vi "Configure Smoothing.vi"(6 "Smoothing Aperture (1.5 %)":dbl=1.5 format="%^#_9g", 7 "Enable Smoothing (Disable)":bool, 8 "error in (no error)":errorcluster, 9 "Select Trace (1: 1)":u16(ring)=1 items=["1"=1, "2"=2, "3"=3, "4"=4, "5"=5, "6"=6, "7"=7, "8"=8], 10 "Measurement Type (6: Phase Noise)":u16(ring)=6 items=["AM Noise"=1, "Baseband Noise"=2, "Freq/Power"=3, "Spectrum"=4, "Transient"=5, "Phase Noise"=6, "User"=7], 11 "VISA resource name":refnum<visa-resource-name>) -> (0 "error out":errorcluster, 3 "VISA resource name out":refnum<visa-resource-name>)   [LabVIEW 2011, in "Agilent E5052X.lvlib"]
doc: "Configures the instrument to apply smoothing to all types of measurement data.\n\n<b>Note: </b>\n\n\"Configure Measurement Characteristics\" VI must be run before this VI."
uses:
  Agilent E5052X.lvlib
panel:
  # "Smoothing Settings"
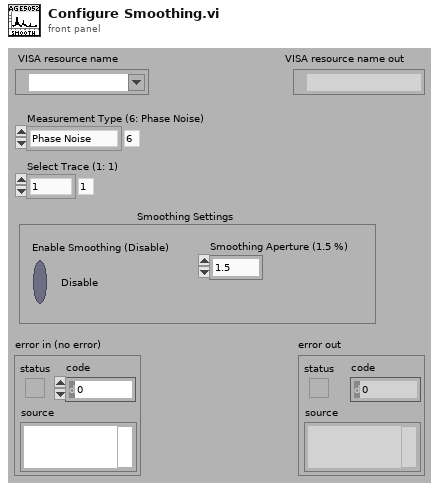
[diagram p1: front panel]
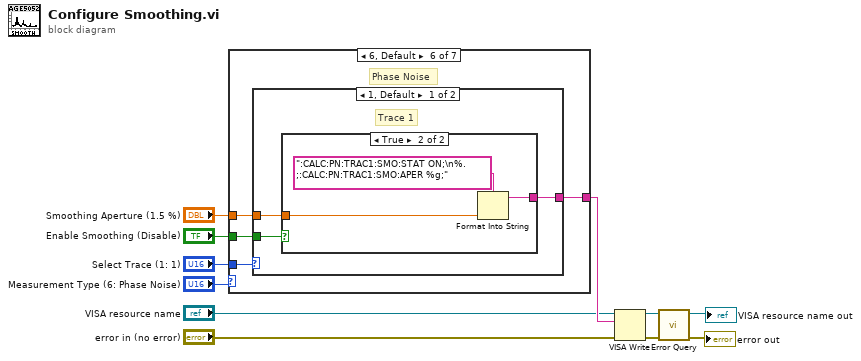
[diagram p0: block diagram]
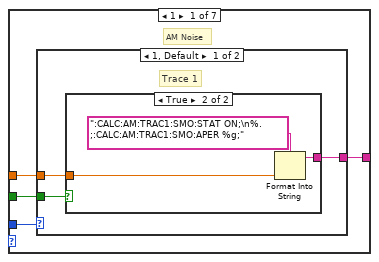
[diagram p2: hidden frame]
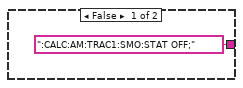
[diagram p3: hidden frame]
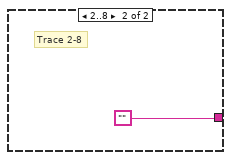
[diagram p4: hidden frame]
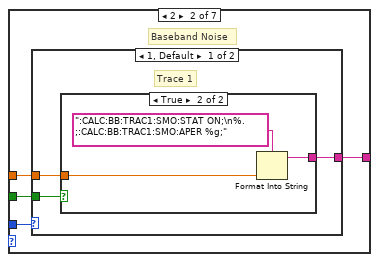
[diagram p5: hidden frame]
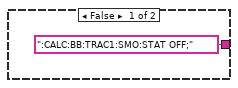
[diagram p6: hidden frame]
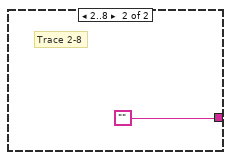
[diagram p7: hidden frame]
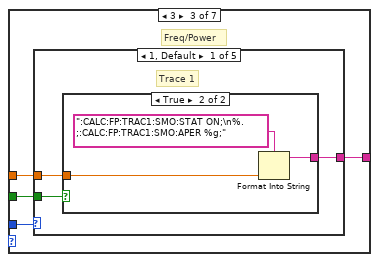
[diagram p8: hidden frame]
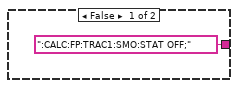
[diagram p9: hidden frame]
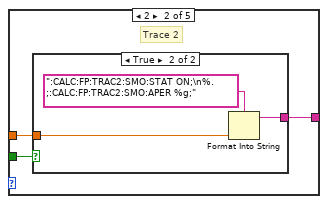
[diagram p10: hidden frame]
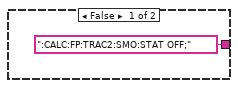
[diagram p11: hidden frame]
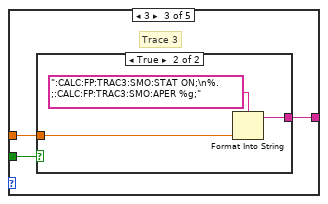
[diagram p12: hidden frame]
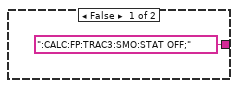
[diagram p13: hidden frame]
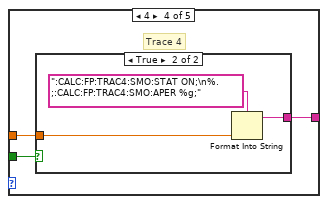
[diagram p14: hidden frame]
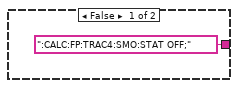
[diagram p15: hidden frame]
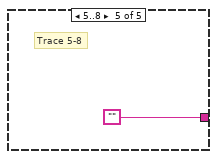
[diagram p16: hidden frame]
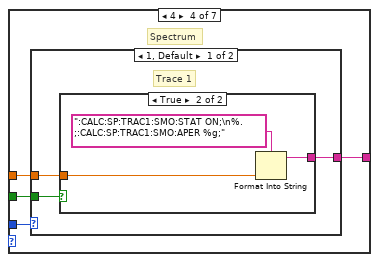
[diagram p17: hidden frame]
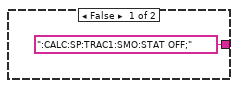
[diagram p18: hidden frame]
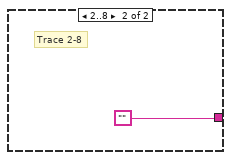
[diagram p19: hidden frame]
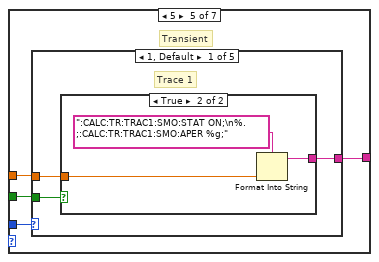
[diagram p20: hidden frame]
diagram:
  n1 = case shown="6, Default" "Measurement Type (6: Phase Noise)" {
    tunnel: "Enable Smoothing (Disable)" -> [w14 w26 w38 w71 w83 w116 w128]
    tunnel: "Select Trace (1: 1)" -> [w15 w25 w37 w70 w82 w115 w127]
    tunnel: "Smoothing Aperture (1.5 %)" -> [w13 w27 w39 w72 w84 w117 w129]
    tunnel: [w12 w24 w36 w69 w81 w114 w126] -> w6
    frame 1 {
      # "AM Noise"
      n2 = case shown="1, Default" w15 {
        tunnel: w14 -> [w18 _]
        tunnel: w13 -> [w17 _]
        tunnel: [w16 ""] -> w12
        frame 1, Default {
          # "Trace 1"
          n3 = case shown="True" w18 {
            tunnel: w17 -> [_ w22]
            tunnel: [":CALC:AM:TRAC1:SMO:STAT OFF;" w20] -> w16
            frame False {
            }
            frame True {
              n4 = Format Into String(format string=":CALC:AM:TRAC1:SMO:STAT ON;\n%.;:CALC:AM:TRAC1:SMO:APER %g;", w22) -> (resulting string=w20:string)  [unwired: 2 in, 1 out]
            }
          }
        }
        frame 2..8 {
          # "Trace 2-8"
        }
      }
    }
    frame 2 {
      # "Baseband Noise"
      n5 = case shown="1, Default" w25 {
        tunnel: w26 -> [w30 _]
        tunnel: w27 -> [w29 _]
        tunnel: [w28 ""] -> w24
        frame 1, Default {
          # "Trace 1"
          n6 = case shown="True" w30 {
            tunnel: w29 -> [_ w34]
            tunnel: [":CALC:BB:TRAC1:SMO:STAT OFF;" w32] -> w28
            frame False {
            }
            frame True {
              n7 = Format Into String(format string=":CALC:BB:TRAC1:SMO:STAT ON;\n%.;:CALC:BB:TRAC1:SMO:APER %g;", w34) -> (resulting string=w32:string)  [unwired: 2 in, 1 out]
            }
          }
        }
        frame 2..8 {
          # "Trace 2-8"
        }
      }
    }
    frame 3 {
      # "Freq/Power"
      n8 = case shown="1, Default" w37 {
        tunnel: w38 -> [w42 w48 w55 w62 _]
        tunnel: w39 -> [w41 w49 w56 w63 _]
        tunnel: [w40 w47 w54 w61 ""] -> w36
        frame 1, Default {
          # "Trace 1"
          n9 = case shown="True" w42 {
            tunnel: w41 -> [_ w46]
            tunnel: [":CALC:FP:TRAC1:SMO:STAT OFF;" w44] -> w40
            frame False {
            }
            frame True {
              n10 = Format Into String(format string=":CALC:FP:TRAC1:SMO:STAT ON;\n%.;:CALC:FP:TRAC1:SMO:APER %g;", w46) -> (resulting string=w44:string)  [unwired: 2 in, 1 out]
            }
          }
        }
        frame 2 {
          # "Trace 2"
          n11 = case shown="True" w48 {
            tunnel: w49 -> [_ w53]
            tunnel: [":CALC:FP:TRAC2:SMO:STAT OFF;" w51] -> w47
            frame False {
            }
            frame True {
              n12 = Format Into String(format string=":CALC:FP:TRAC2:SMO:STAT ON;\n%.;:CALC:FP:TRAC2:SMO:APER %g;", w53) -> (resulting string=w51:string)  [unwired: 2 in, 1 out]
            }
          }
        }
        frame 3 {
          # "Trace 3"
          n13 = case shown="True" w55 {
            tunnel: w56 -> [_ w60]
            tunnel: [":CALC:FP:TRAC3:SMO:STAT OFF;" w58] -> w54
            frame False {
            }
            frame True {
              n14 = Format Into String(format string=":CALC:FP:TRAC3:SMO:STAT ON;\n%.;:CALC:FP:TRAC3:SMO:APER %g;", w60) -> (resulting string=w58:string)  [unwired: 2 in, 1 out]
            }
          }
        }
        frame 4 {
          # "Trace 4"
          n15 = case shown="True" w62 {
            tunnel: w63 -> [_ w67]
            tunnel: [":CALC:FP:TRAC4:SMO:STAT OFF;" w65] -> w61
            frame False {
            }
            frame True {
              n16 = Format Into String(format string=":CALC:FP:TRAC4:SMO:STAT ON;\n%.;:CALC:FP:TRAC4:SMO:APER %g;", w67) -> (resulting string=w65:string)  [unwired: 2 in, 1 out]
            }
          }
        }
        frame 5..8 {
          # "Trace 5-8"
        }
      }
    }
    frame 4 {
      # "Spectrum"
      n17 = case shown="1, Default" w70 {
        tunnel: w71 -> [w75 _]
        tunnel: w72 -> [w74 _]
        tunnel: [w73 ""] -> w69
        frame 1, Default {
          # "Trace 1"
          n18 = case shown="True" w75 {
            tunnel: w74 -> [_ w79]
            tunnel: [":CALC:SP:TRAC1:SMO:STAT OFF;" w77] -> w73
            frame False {
            }
            frame True {
              n19 = Format Into String(format string=":CALC:SP:TRAC1:SMO:STAT ON;\n%.;:CALC:SP:TRAC1:SMO:APER %g;", w79) -> (resulting string=w77:string)  [unwired: 2 in, 1 out]
            }
          }
        }
        frame 2..8 {
          # "Trace 2-8"
        }
      }
    }
    frame 5 {
      # "Transient"
      n20 = case shown="1, Default" w82 {
        tunnel: w83 -> [w87 w93 w100 w107 _]
        tunnel: w84 -> [w86 w94 w101 w108 _]
        tunnel: [w85 w92 w99 w106 ""] -> w81
        frame 1, Default {
          # "Trace 1"
          n21 = case shown="True" w87 {
            tunnel: w86 -> [_ w91]
            tunnel: [":CALC:TR:TRAC1:SMO:STAT OFF;" w89] -> w85
            frame False {
            }
            frame True {
              n22 = Format Into String(format string=":CALC:TR:TRAC1:SMO:STAT ON;\n%.;:CALC:TR:TRAC1:SMO:APER %g;", w91) -> (resulting string=w89:string)  [unwired: 2 in, 1 out]
            }
          }
        }
        frame 2 {
          # "Trace 2"
          n23 = case shown="True" w93 {
            tunnel: w94 -> [_ w98]
            tunnel: [":CALC:TR:TRAC2:SMO:STAT OFF;" w96] -> w92
            frame False {
            }
            frame True {
              n24 = Format Into String(format string=":CALC:TR:TRAC2:SMO:STAT ON;\n%.;:CALC:TR:TRAC2:SMO:APER %g;", w98) -> (resulting string=w96:string)  [unwired: 2 in, 1 out]
            }
          }
        }
        frame 3 {
          # "Trace 3"
          n25 = case shown="True" w100 {
            tunnel: w101 -> [_ w105]
            tunnel: [":CALC:TR:TRAC3:SMO:STAT OFF;" w103] -> w99
            frame False {
            }
            frame True {
              n26 = Format Into String(format string=":CALC:TR:TRAC3:SMO:STAT ON;\n%.;:CALC:TR:TRAC3:SMO:APER %g;", w105) -> (resulting string=w103:string)  [unwired: 2 in, 1 out]
            }
          }
        }
        frame 4 {
          # "Trace 4"
          n27 = case shown="True" w107 {
            tunnel: w108 -> [_ w112]
            tunnel: [":CALC:TR:TRAC4:SMO:STAT OFF;" w110] -> w106
            frame False {
            }
            frame True {
              n28 = Format Into String(format string=":CALC:TR:TRAC4:SMO:STAT ON;\n%.;:CALC:TR:TRAC4:SMO:APER %g;", w112) -> (resulting string=w110:string)  [unwired: 2 in, 1 out]
            }
          }
        }
        frame 5..8 {
          # "Trace 5-8"
        }
      }
    }
    frame 6, Default {
      # "Phase Noise"
      n29 = case shown="1, Default" w115 {
        tunnel: w116 -> [w120 _]
        tunnel: w117 -> [w119 _]
        tunnel: [w118 ""] -> w114
        frame 1, Default {
          # "Trace 1"
          n30 = case shown="True" w120 {
            tunnel: w119 -> [_ w124]
            tunnel: [":CALC:PN:TRAC1:SMO:STAT OFF;" w122] -> w118
            frame False {
            }
            frame True {
              n31 = Format Into String(format string=":CALC:PN:TRAC1:SMO:STAT ON;\n%.;:CALC:PN:TRAC1:SMO:APER %g;", w124) -> (resulting string=w122:string)  [unwired: 2 in, 1 out]
            }
          }
        }
        frame 2..8 {
          # "Trace 2-8"
        }
      }
    }
    frame 7 {
      # "User"
      n32 = case shown="1, Default" w127 {
        tunnel: w128 -> [w132 w138 w145 w152 w159 w166 w173 w180]
        tunnel: w129 -> [w131 w139 w146 w153 w160 w167 w174 w181]
        tunnel: [w130 w137 w144 w151 w158 w165 w172 w179] -> w126
        frame 1, Default {
          # "Trace 1"
          n33 = case shown="True" w132 {
            tunnel: w131 -> [_ w136]
            tunnel: [":CALC:USER:TRAC1:SMO:STAT OFF;" w134] -> w130
            frame False {
            }
            frame True {
              n34 = Format Into String(format string=":CALC:USER:TRAC1:SMO:STAT ON;\n%.;:CALC:USER:TRAC1:SMO:APER %g;", w136) -> (resulting string=w134:string)  [unwired: 2 in, 1 out]
            }
          }
        }
        frame 2 {
          # "Trace 2"
          n35 = case shown="True" w138 {
            tunnel: w139 -> [_ w143]
            tunnel: [":CALC:USER:TRAC2:SMO:STAT OFF;" w141] -> w137
            frame False {
            }
            frame True {
              n36 = Format Into String(format string=":CALC:USER:TRAC2:SMO:STAT ON;\n%.;:CALC:USER:TRAC2:SMO:APER %g;", w143) -> (resulting string=w141:string)  [unwired: 2 in, 1 out]
            }
          }
        }
        frame 3 {
          # "Trace 3"
          n37 = case shown="True" w145 {
            tunnel: w146 -> [_ w150]
            tunnel: [":CALC:USER:TRAC3:SMO:STAT OFF;" w148] -> w144
            frame False {
            }
            frame True {
              n38 = Format Into String(format string=":CALC:USER:TRAC3:SMO:STAT ON;\n%.;:CALC:USER:TRAC3:SMO:APER %g;", w150) -> (resulting string=w148:string)  [unwired: 2 in, 1 out]
            }
          }
        }
        frame 4 {
          # "Trace 4"
          n39 = case shown="True" w152 {
            tunnel: w153 -> [_ w157]
            tunnel: [":CALC:USER:TRAC4:SMO:STAT OFF;" w155] -> w151
            frame False {
            }
            frame True {
              n40 = Format Into String(format string=":CALC:USER:TRAC4:SMO:STAT ON;\n%.;:CALC:USER:TRAC4:SMO:APER %g;", w157) -> (resulting string=w155:string)  [unwired: 2 in, 1 out]
            }
          }
        }
        frame 5 {
          # "Trace 5"
          n41 = case shown="True" w159 {
            tunnel: w160 -> [_ w164]
            tunnel: [":CALC:USER:TRAC5:SMO:STAT OFF;" w162] -> w158
            frame False {
            }
            frame True {
              n42 = Format Into String(format string=":CALC:USER:TRAC5:SMO:STAT ON;\n%.;:CALC:USER:TRAC5:SMO:APER %g;", w164) -> (resulting string=w162:string)  [unwired: 2 in, 1 out]
            }
          }
        }
        frame 6 {
          # "Trace 6"
          n43 = case shown="True" w166 {
            tunnel: w167 -> [_ w171]
            tunnel: [":CALC:USER:TRAC6:SMO:STAT OFF;" w169] -> w165
            frame False {
            }
            frame True {
              n44 = Format Into String(format string=":CALC:USER:TRAC6:SMO:STAT ON;\n%.;:CALC:USER:TRAC6:SMO:APER %g;", w171) -> (resulting string=w169:string)  [unwired: 2 in, 1 out]
            }
          }
        }
        frame 7 {
          # "Trace 7"
          n45 = case shown="True" w173 {
            tunnel: w174 -> [_ w178]
            tunnel: [":CALC:USER:TRAC7:SMO:STAT OFF;" w176] -> w172
            frame False {
            }
            frame True {
              n46 = Format Into String(format string=":CALC:USER:TRAC7:SMO:STAT ON;\n%.;:CALC:USER:TRAC7:SMO:APER %g;", w178) -> (resulting string=w176:string)  [unwired: 2 in, 1 out]
            }
          }
        }
        frame 8 {
          # "Trace 8"
          n47 = case shown="True" w180 {
            tunnel: w181 -> [_ w185]
            tunnel: [":CALC:USER:TRAC8:SMO:STAT OFF;" w183] -> w179
            frame False {
            }
            frame True {
              n48 = Format Into String(format string=":CALC:USER:TRAC8:SMO:STAT ON;\n%.;:CALC:USER:TRAC8:SMO:APER %g;", w185) -> (resulting string=w183:string)  [unwired: 2 in, 1 out]
            }
          }
        }
      }
    }
  }
  n49 = VISA Write(VISA resource name="VISA resource name", write buffer=w6, error in (no error)="error in (no error)") -> (VISA resource name out=w7:refnum<visa-resource-name>, error out=w8:errorcluster)  [unwired: 1 out]
  n50 = call "Error Query.vi"("error in (no error)"=w8, "VISA resource name"=w7) -> ("error out"=→"error out":errorcluster, "VISA resource name out"=→"VISA resource name out":refnum<visa-resource-name>)  [unwired: 6 in, 2 out]
